vi "GoogleMapsAPI_V2009.vi"() -> ()   [LabVIEW 2019]
uses:
  <userlib>/ROS for LabVIEW Software/ROS/Code/Console/Servers/ServerSubs/TopicDef.ctl
  <userlib>/ROS for LabVIEW Software/ROS/Code/SubVIs/_ROSDirection.ctl
  <userlib>/ROS for LabVIEW Software/ROS/MessageParsing/std_msgs/subs/parse_float32_scalar.vi
panel:
  out "Longitude":dbl
  out "Latitude":dbl
  in  "stop":bool
  in  "Google Maps API Key":string
  in  "character":string="a"
  in  "color":string(combo)="purple"
  in  "size":string(combo)="mid"
  in  "Map Format":string(combo)="hybrid"
  in  "X":dbl=350.0
  in  "Y":dbl=570.0
  in  "Zoom":sgl=18.0 format="%#.1g"
  out "URL":string="http://maps.google.com/staticmap?center=51.406200,-1.307000&zoom=18&size=570x350&maptype=hybrid&markers=51.406200,-1.307000,midpurplea&key=&path=rgb:0xFF1000,weight:5|51.406200,-1.307000|51.406200,-1.307000"
  in  "?":refnum<k7>(container)
  # "Balloon Position"
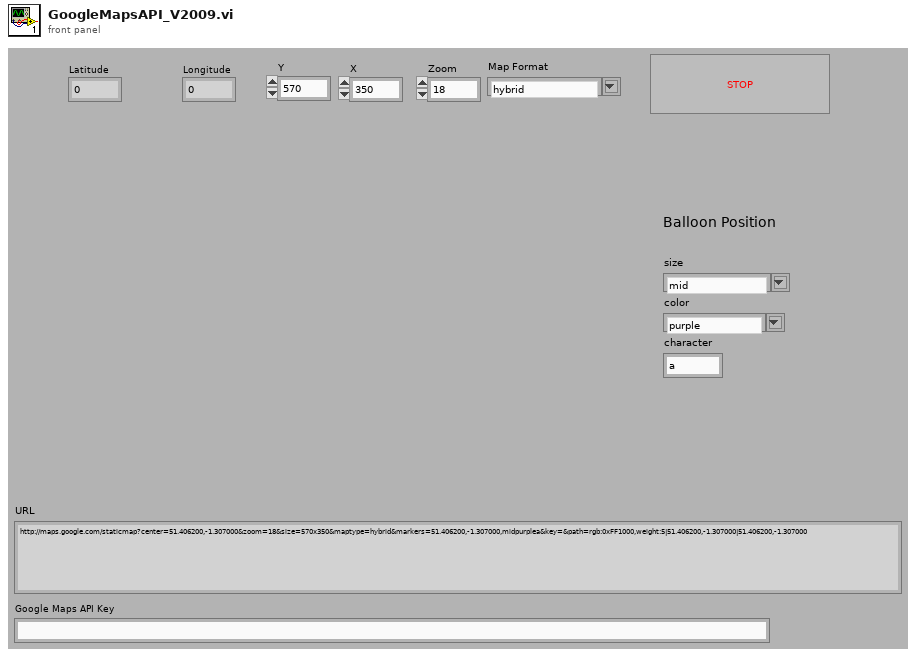
[diagram p1: front panel]
types:
  T1 = typedef "TopicDef.ctl" = cluster{"Topic":string, "Type":string, "Action":T2, "Update (ms)":u16, "queue size":u16}
  T2 = typedef "_ROSDirection.ctl" = enum16{"Node", "Publisher", "Subscriber", "ServiceClient", "ServiceProvider"}
  T3 = typedef "_ROSControl.ctl" = cluster{"topic port":u16, "Node":string, "topic":string, "type":string, "node port":u16, "error ":errorcluster, "Direction":T2, "Update (ms)":u16, "FIFO size":u16}
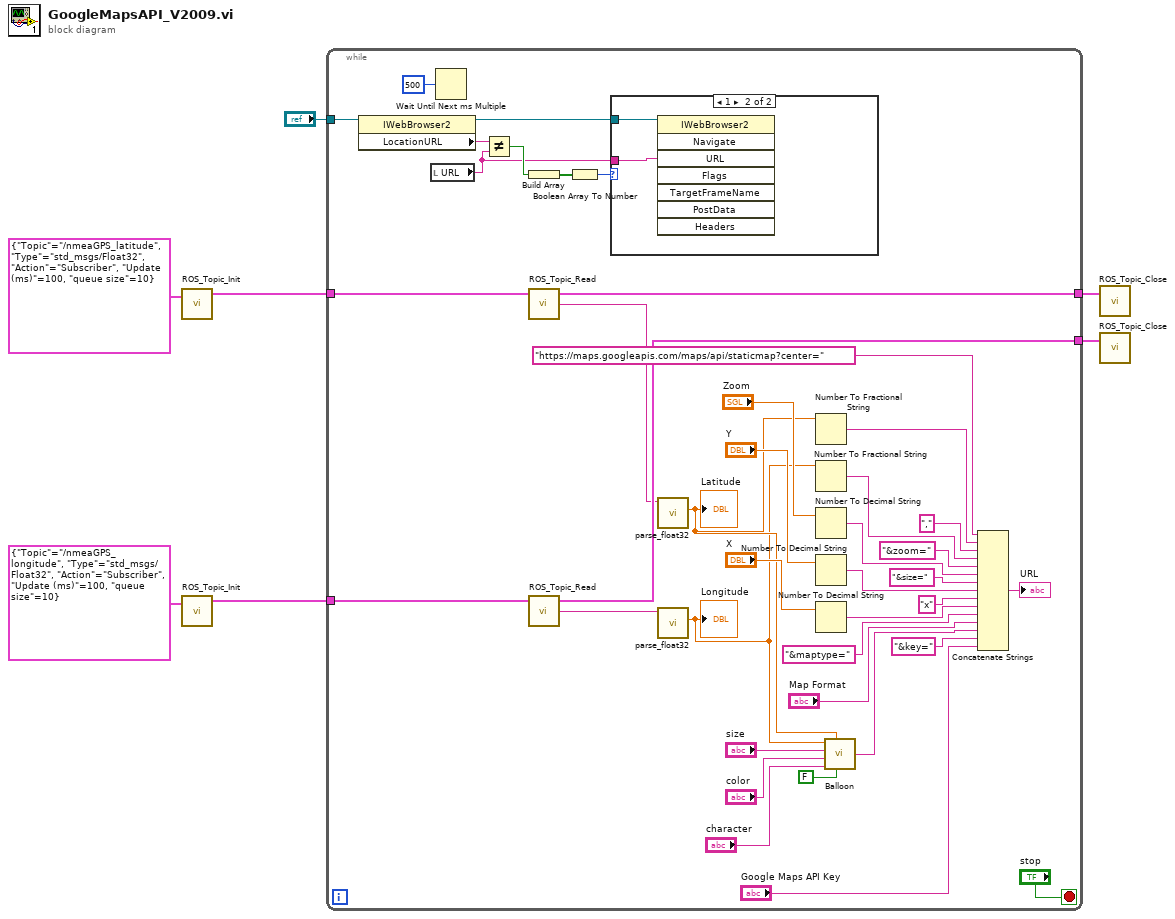
[diagram p0: block diagram]
diagram:
  n1 = call <userlib>:"ROS_Topic_Init.vi"("Definitions"=T1 {"Topic"="/nmeaGPS_latitude", "Type"="std_msgs/Float32", "Action"=enum."Subscriber", "Update (ms)"=100, "queue size"=10}) -> ("ROS out"=w2:T3)  [unwired: 2 in, 1 out]
  n2 = call <userlib>:"ROS_Topic_Init.vi"("Definitions"=T1 {"Topic"="/nmeaGPS_longitude", "Type"="std_msgs/Float32", "Action"=enum."Subscriber", "Update (ms)"=100, "queue size"=10}) -> ("ROS out"=w4:T3)  [unwired: 2 in, 1 out]
  n3 = while {
    tunnel: "?" -> [w46]
    tunnel: w4 -> [w15]
    tunnel: [w14] -> w3
    tunnel: w2 -> [w12]
    tunnel: [w11] -> w1
    stop <- "stop" stop-if-true
    n4 = property class="IWebBrowser2"(reference=w46) -> (reference out=w45:refnum<k7>, "LocationURL"=w43:string)  [unwired: 1 in, 1 out]
    n5 = local read "URL"() -> (w40:string)
    n6 = Wait Until Next ms Multiple(millisecond multiple=u32 500) -> ()  [unwired: 1 out]
    n7 = Not Equal?(x=w43, y=w40) -> (x != y?=w44:bool)
    n8 = Build Array(w44) -> (w42:bool[])
    n9 = call <userlib>:"ROS_Topic_Read.vi"("ROS in"=w12) -> ("Reply"=w13:string, "ROS out"=w11:T3)  [unwired: 2 in, 1 out]
    n10 = call <userlib>:"ROS_Topic_Read.vi"("ROS in"=w15) -> ("Reply"=w16:string, "ROS out"=w14:T3)  [unwired: 2 in, 1 out]
    n11 = Boolean Array To Number(Boolean array=w42) -> (number=w41:u32)
    n12 = case shown="1" w41 {
      tunnel: w40 -> [_ w49]
      tunnel: w45 -> [_ w48]
      frame 0, Default {
      }
      frame 1 {
        n13 = invoke class="IWebBrowser2" method="Navigate"(reference=w48, "URL"=w49) -> ()  [unwired: 6 in, 8 out]
      }
    }
    n14 = call-poly <userlib>:"parse_float32.vi"("msg in"=w13) -> ("number"=w10:sgl)  [unwired: 4 in, 2 out]
    "Latitude" <- w10
    n15 = call-poly <userlib>:"parse_float32.vi"("msg in"=w16) -> ("number"=w9:sgl)  [unwired: 4 in, 2 out]
    "Longitude" <- w9
    n16 = Number To Fractional String(number=w10) -> (F-format string=w21:string)  [unwired: 3 in]
    n17 = Number To Fractional String(number=w9) -> (F-format string=w20:string)  [unwired: 3 in]
    n18 = Number To Decimal String(number="Zoom") -> (decimal integer string=w35:string)  [unwired: 1 in]
    n19 = Number To Decimal String(number="Y") -> (decimal integer string=w31:string)  [unwired: 1 in]
    n20 = Number To Decimal String(number="X") -> (decimal integer string=w29:string)  [unwired: 1 in]
    n21 = call "Balloon.vi"("One more?"=FALSE, "Latitude"=w10, "Character"="character", "Color"="color", "Size"="size", "Longitude"=w9) -> ("Balloon"=w26:string)
    n22 = Concatenate Strings("https://maps.googleapis.com/maps/api/staticmap?center=" ("URL"), w21, "," ("string"), w20, "&zoom=", w35, "&size=", w31, "x", w29, "&maptype=", "Map Format", w26, "&key=" ("string"), "Google Maps API Key") -> (→"URL":string)
  }
  n23 = call <userlib>:"ROS_Topic_Close.vi"("ROS in"=w1) -> ()  [unwired: 3 in, 1 out]
  n24 = call <userlib>:"ROS_Topic_Close.vi"("ROS in"=w3) -> ()  [unwired: 3 in, 1 out]
